vi "Mode_Ref_API.vi"(0 "DVR In":refnum<data-value>, 11 "Error In":errorcluster) -> (4 "DVR Out":refnum<data-value>, 6 "VI Ref":refnum<vi>, 15 "Error out":errorcluster)   [LabVIEW 2020, in "Test.lvclass"]
doc: "Mode Reference API"
uses:
  Test.lvclass
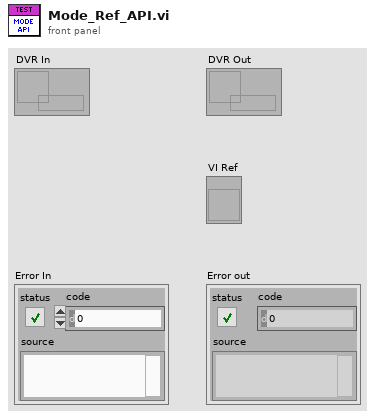
[diagram p1: front panel]
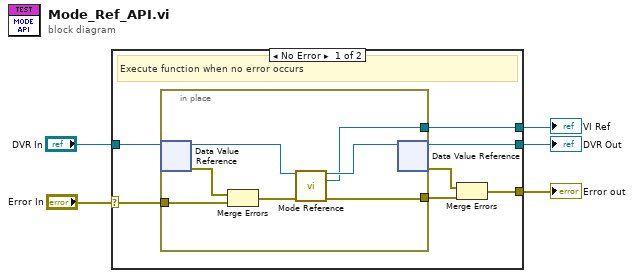
[diagram p0: block diagram]
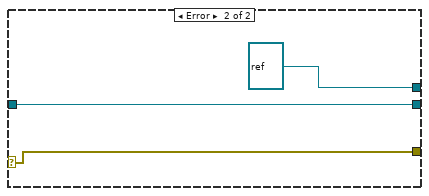
[diagram p2: hidden frame]
diagram:
  n1 = case shown="No Error" "Error In" {
    selector: "Error In" -> [w12 w20]
    tunnel: "DVR In" -> [w11 w21]
    tunnel: [w10 w21] -> w3
    tunnel: [w6 w20] -> w2
    tunnel: [w9 refnum<vi> refnum ("VI Refnum")] -> w1
    frame No Error {
      # "Execute function when no error occurs"
      n2 = in-place {
        in-place-border: w12 -> [w19]
        in-place-border: [w15] -> w8
        in-place-border: [w13] -> w9
        n3 = in-place-dvr #1(w11) -> (w16:refnum<class "Test.lvclass">, w18:errorcluster)
        n4 = Merge Errors(w18, w19) -> (w17:errorcluster)
        n5 = call-dynamic "Mode Reference.vi"("Test in"=w16, "Error in"=w17) -> ("Test out"=w14:refnum<class "Test.lvclass">, "VI Refnum"=w13:refnum<vi>, "Error out"=w15:errorcluster)  [unwired: 11 in]
        n6 = in-place-dvr #1(w14) -> (w10:refnum<data-value>, w7:errorcluster)
      }
      n7 = Merge Errors(w7, w8) -> (w6:errorcluster)
    }
    frame Error {
    }
  }
  "DVR Out" <- w3
  "Error out" <- w2
  "VI Ref" <- w1
